vi "build InteractionParameterReceived payload.vi"(9 "data":u8[](array[numeric]), 10 "parameterHandle in":u64, 11 "interactionClassHandle":u64) -> (3 "interaction_attribute_type":T1)   [LabVIEW 2019, in "HLA Custom Device Engine.lvlib"]
uses:
  HLA Custom Device Engine.lvlib
  _typedefs/interaction_attribute_received_type.ctl
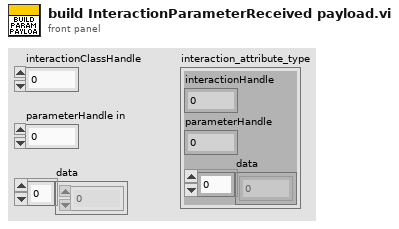
[diagram p1: front panel]
types:
  T1 = typedef "HLA Custom Device Engine.lvlib/interaction_attribute_received_type.ctl" = cluster{"interactionHandle":u64, "parameterHandle":u64, "data":u8[]}
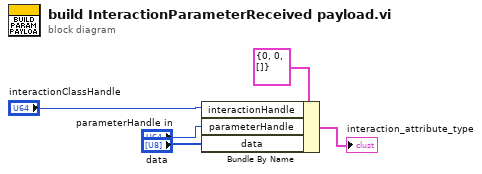
[diagram p0: block diagram]
diagram:
  n1 = Bundle By Name(cluster=T1 {"interactionHandle"=0, "parameterHandle"=0, "data"=[]}, "interactionHandle"="interactionClassHandle", "parameterHandle"="parameterHandle in", "data"="data") -> (→"interaction_attribute_type":T1)
